vi "DM65-Tutorial-3.vi"() -> ()   [LabVIEW 2020]
uses:
  C:/TwinCAT/AdsApi/.NET/v4.0.30319/TwinCAT.Ads.dll
  TwinCAT/AdsApi/.NET/v4.0.30319/TwinCAT.Ads.dll
panel:
  out "MDN":bool
  out "FDN":bool
  out "FUP":bool
  out "MUP":bool
  out "box":bool
  in  "fotocellula":bool
  in  "sensore":bool
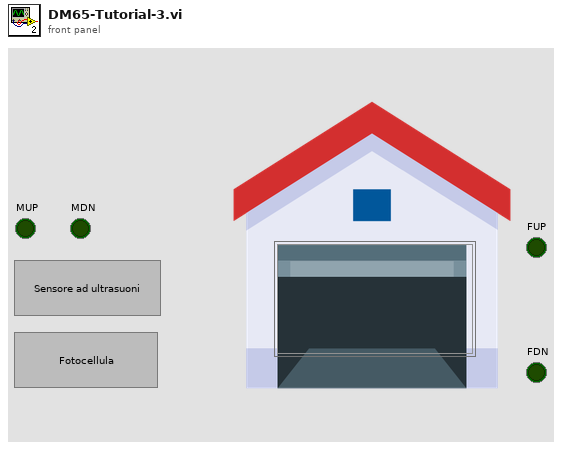
[diagram p1: front panel]
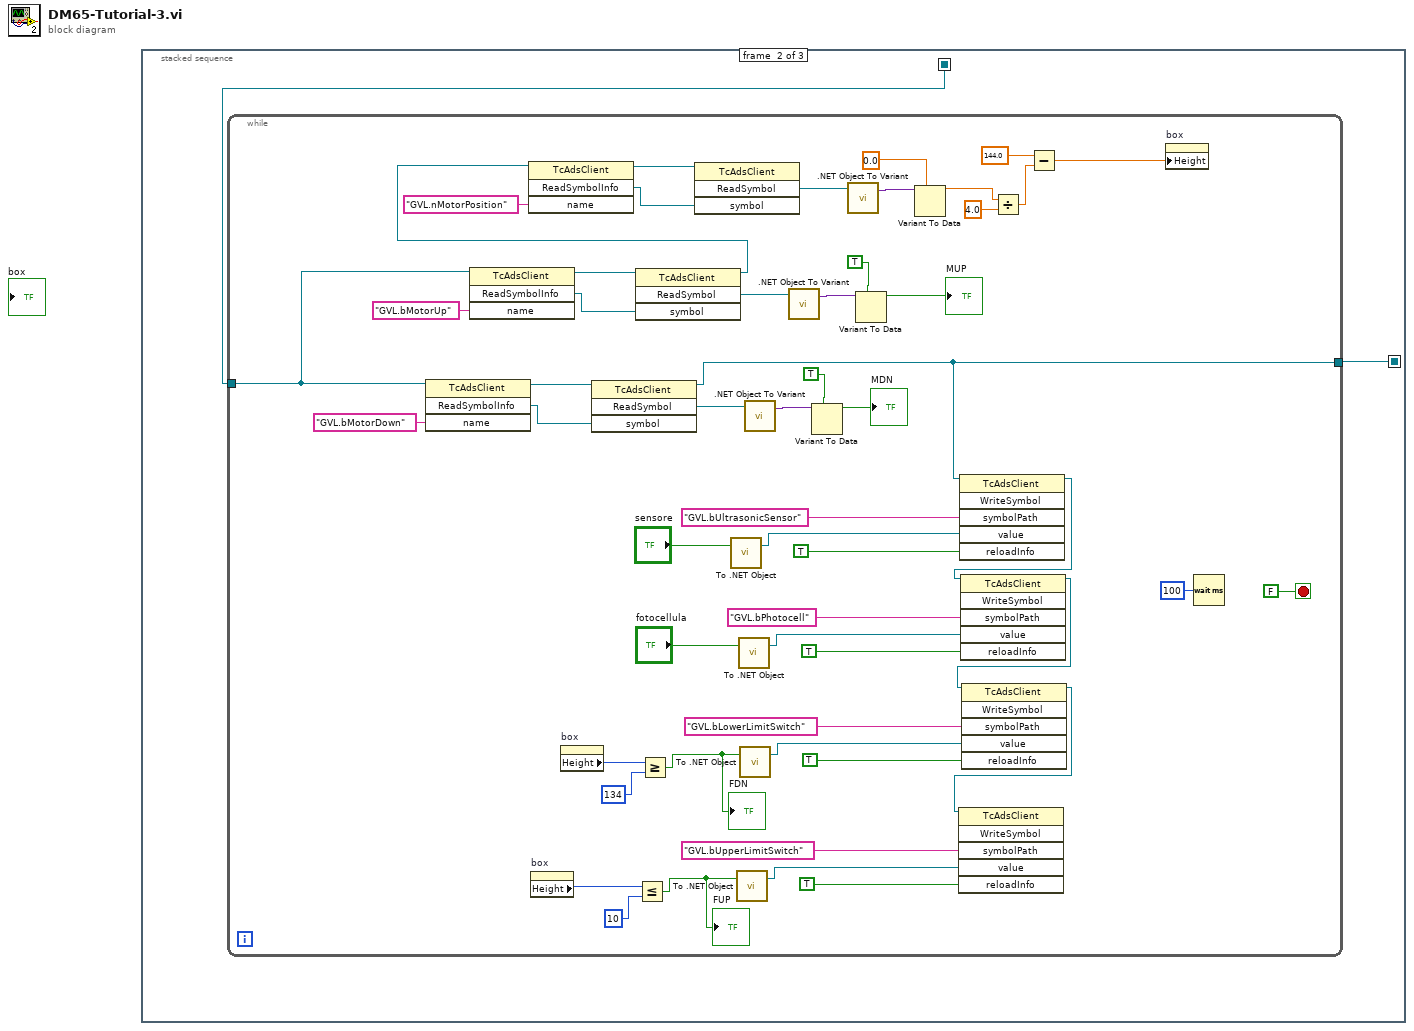
[diagram p0: block diagram]
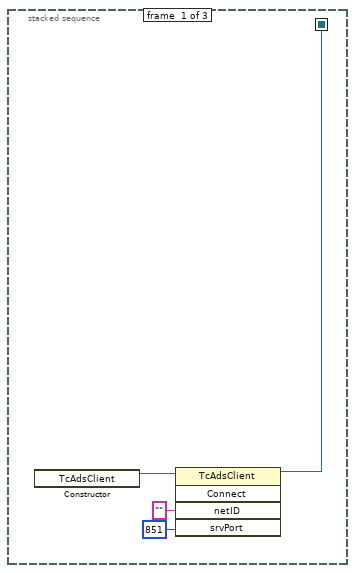
[diagram p2: hidden frame]
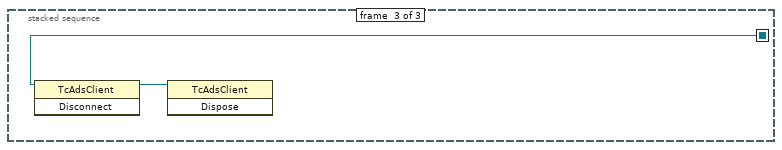
[diagram p3: hidden frame]
diagram:
  n1 = stacked-sequence {
    seq-local: [w1 _ _] -> [_ w6 _]
    seq-local: [_ w5 _] -> [_ _ w61]
    frame #0 {
      n2 = constructor class="TcAdsClient"() -> (reference out=w4:refnum<k24>)  [unwired: 3 in, 2 out]
      n3 = invoke class="TcAdsClient" method="Connect"(reference=w4, "netID"="", "srvPort"=851) -> (reference out=w1:refnum<k24>)  [unwired: 2 in, 4 out]
    }
    frame #1 {
      n4 = while {
        tunnel: w6 -> [w22]
        tunnel: [w30] -> w5
        stop <- FALSE stop-if-true
        n5 = invoke class="TcAdsClient" method="ReadSymbolInfo"(reference=w22, "name"="GVL.bMotorDown") -> (reference out=w57:refnum<k24>, "ReadSymbolInfo"=w56:refnum<k24>)  [unwired: 2 in, 2 out]
        n6 = invoke class="TcAdsClient" method="ReadSymbolInfo"(reference=w22, "name"="GVL.bMotorUp") -> (reference out=w27:refnum<k24>, "ReadSymbolInfo"=w26:refnum<k24>)  [unwired: 2 in, 2 out]
        n7 = property on="box" class="Bool (strict)"() -> ("Height"=w33:u32)  [unwired: 2 in, 2 out]
        n8 = property on="box" class="Bool (strict)"() -> ("Height"=w40:u32)  [unwired: 2 in, 2 out]
        n9 = invoke class="TcAdsClient" method="ReadSymbol"(reference=w57, "symbol"=w56) -> (reference out=w30:refnum<k24>, "ReadSymbol"=w55:refnum<k24>)  [unwired: 2 in, 2 out]
        n10 = invoke class="TcAdsClient" method="ReadSymbol"(reference=w27, "symbol"=w26) -> (reference out=w15:refnum<k24>, "ReadSymbol"=w25:refnum<k24>)  [unwired: 2 in, 2 out]
        n11 = invoke class="TcAdsClient" method="ReadSymbolInfo"(reference=w15, "name"="GVL.nMotorPosition") -> (reference out=w19:refnum<k24>, "ReadSymbolInfo"=w18:refnum<k24>)  [unwired: 2 in, 2 out]
        n12 = Less Or Equal?(x=w33, y=u32 10) -> (x <= y?=w13:bool)
        "FUP" <- w13
        n13 = Greater Or Equal?(x=w40, y=u32 134) -> (x >= y?=w14:bool)
        "FDN" <- w14
        n14 = invoke class="TcAdsClient" method="ReadSymbol"(reference=w19, "symbol"=w18) -> ("ReadSymbol"=w17:refnum<k24>)  [unwired: 2 in, 3 out]
        n15 = call <vilib>:"To .NET Object.vi"("anything"="sensore") -> (".NET object"=w49:refnum<k24>)  [unwired: 1 in, 1 out]
        n16 = call <vilib>:"To .NET Object.vi"("anything"=w13) -> (".NET object"=w36:refnum<k24>)  [unwired: 1 in, 1 out]
        n17 = call <vilib>:"To .NET Object.vi"("anything"="fotocellula") -> (".NET object"=w46:refnum<k24>)  [unwired: 1 in, 1 out]
        n18 = call <vilib>:"To .NET Object.vi"("anything"=w14) -> (".NET object"=w42:refnum<k24>)  [unwired: 1 in, 1 out]
        n19 = call <vilib>:".NET Object To Variant.vi"(".NET object"=w55) -> ("variant"=w54:variant)  [unwired: 1 in, 1 out]
        n20 = call <vilib>:".NET Object To Variant.vi"(".NET object"=w25) -> ("variant"=w24:variant)  [unwired: 1 in, 1 out]
        n21 = Variant To Data(type=TRUE, Variant=w54) -> (data=→"MDN":bool)  [unwired: 1 in, 1 out]
        n22 = call <vilib>:".NET Object To Variant.vi"(".NET object"=w17) -> ("variant"=w16:variant)  [unwired: 1 in, 1 out]
        n23 = Variant To Data(type=TRUE, Variant=w24) -> (data=→"MUP":bool)  [unwired: 1 in, 1 out]
        n24 = Variant To Data(type=0.0, Variant=w16) -> (data=w12:dbl)  [unwired: 1 in, 1 out]
        n25 = invoke class="TcAdsClient" method="WriteSymbol"(reference=w30, "symbolPath"="GVL.bUltrasonicSensor", "value"=w49, "reloadInfo"=TRUE) -> (reference out=w31:refnum<k24>)  [unwired: 2 in, 5 out]
        n26 = invoke class="TcAdsClient" method="WriteSymbol"(reference=w31, "symbolPath"="GVL.bPhotocell", "value"=w46, "reloadInfo"=TRUE) -> (reference out=w38:refnum<k24>)  [unwired: 2 in, 5 out]
        n27 = invoke class="TcAdsClient" method="WriteSymbol"(reference=w38, "symbolPath"="GVL.bLowerLimitSwitch", "value"=w42, "reloadInfo"=TRUE) -> (reference out=w32:refnum<k24>)  [unwired: 2 in, 5 out]
        n28 = invoke class="TcAdsClient" method="WriteSymbol"(reference=w32, "symbolPath"="GVL.bUpperLimitSwitch", "value"=w36, "reloadInfo"=TRUE) -> ()  [unwired: 2 in, 6 out]
        n29 = Divide(x=w12, y=4.0) -> (x/y=w8:dbl)
        n30 = Subtract(x=144.0, y=w8) -> (x-y=w9:dbl)
        n31 = property on="box" class="Bool (strict)"("Height"=w9) -> ()  [unwired: 2 in, 2 out]
        n32 = Wait (ms)(milliseconds to wait=u32 100) -> ()  [unwired: 1 out]
      }
    }
    frame #2 {
      n33 = invoke class="TcAdsClient" method="Disconnect"(reference=w61) -> (reference out=w60:refnum<k24>)  [unwired: 2 in, 2 out]
      n34 = invoke class="TcAdsClient" method="Dispose"(reference=w60) -> ()  [unwired: 2 in, 3 out]
    }
  }
